vi "Add Channel to Objects.vi"(8 "error in":errorcluster, 9 "Add? (T)":bool=TRUE, 10 "Line Item in":T1, 11 "Objects in":T2) -> (0 "error out":errorcluster, 2 "Line Index":i32)   [LabVIEW 2015, in "TDMS datalogger editor node.lvclass"]
uses:
  TDMS datalogger editor node.lvclass
  <vilib>/NI/DCAF/Tag Editor Core/Table API/Table Manager/object ref.ctl
  <vilib>/NI/DCAF/Tag Editor Core/Configuration Editor/Classes/Engine Parent/Engine Parent Editor Node.lvclass
  <vilib>/NI/DCAF/Tag Editor Core/Configuration Editor/Classes/Module editor node/module editor node.lvclass
  <vilib>/NI/Tag Bus Module Framework/channel/TBM channel.lvclass
  module/configuration/TDMS datalogger configuration.lvclass
  <vilib>/NI/Configuration Framework/serializable configuration/NISE_CEF_serializable configuration.lvclass/NISE_CEF_serializable configuration.ctl
  <vilib>/Utility/LVClass/Get LV Class Name.vi
  <vilib>/NI/Configuration Framework/error generator/NISE_error generator.vi
  <vilib>/NI/Configuration Framework/serializable configuration/NISE_CEF_serializable configuration.lvclass
  <vilib>/NI/DCAF/Tag Editor Core/Table API/Table Manager/Table Manager.lvclass
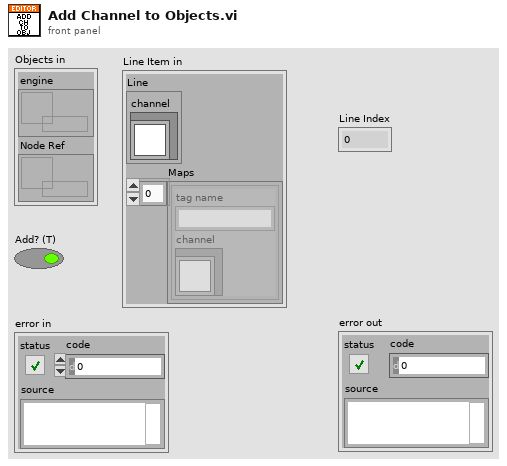
[diagram p1: front panel]
types:
  T1 = cluster{"Line":cluster{"channel":refnum<class "TBM channel.lvclass">}, "Maps":cluster{"tag name":string, "channel":refnum<class "TBM channel.lvclass">}[]}
  T2 = typedef "Table Manager.lvlib/Table Manager.lvclass/object ref.ctl" = cluster{"engine":refnum<data-value>, "Node Ref":refnum<data-value>}
  T3 = cluster{"tag name":string, "channel":refnum<class "TBM channel.lvclass">}[]
  T4 = cluster{"channel":refnum<class "TBM channel.lvclass">}
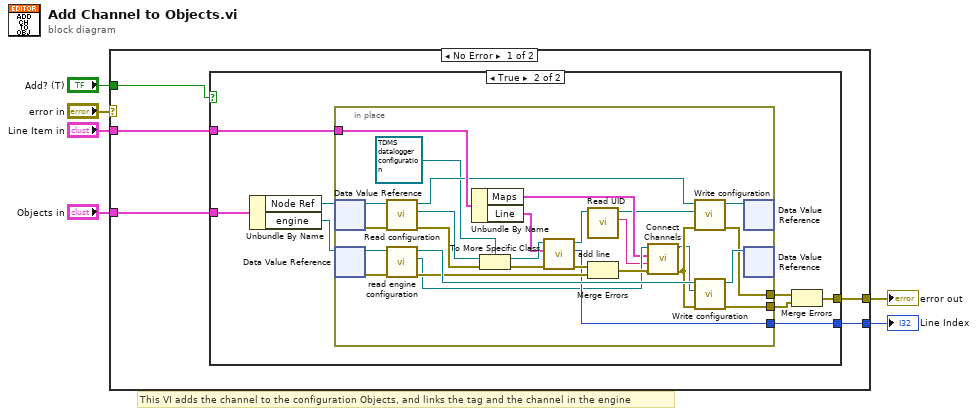
[diagram p0: block diagram]
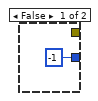
[diagram p2: hidden frame]
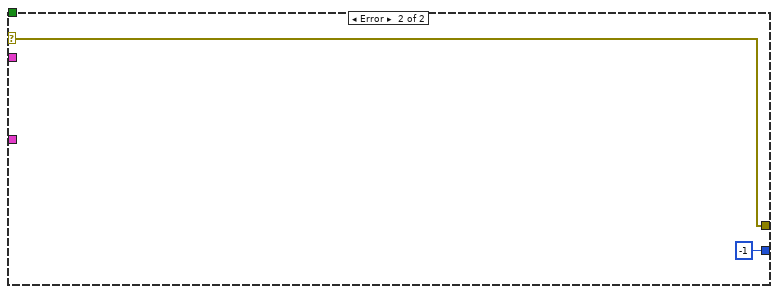
[diagram p3: hidden frame]
diagram:
  # "This VI adds the channel to the configuration Objects, and links the tag and the channel in the engine"
  n1 = case shown="No Error" "error in" {
    selector: "error in" -> [_ w50]
    tunnel: "Objects in" -> [w11 _]
    tunnel: "Line Item in" -> [w10 _]
    tunnel: "Add? (T)" -> [w9 _]
    tunnel: [w8 w50] -> w3
    tunnel: [w7 -1 ("Line Index")] -> w2
    frame No Error {
      n2 = case shown="True" w9 {
        tunnel: [_ w18] -> w8
        tunnel: w10 -> [_ w20]
        tunnel: w11 -> [_ w19]
        tunnel: [-1 ("Line Index") w13] -> w7
        frame False {
        }
        frame True {
          n3 = Unbundle By Name(w19) -> ("Node Ref"=w17:refnum<data-value>, "engine"=w16:refnum<data-value>)
          n4 = in-place {
            in-place-border: w20 -> [w48]
            in-place-border: [w41] -> w15
            in-place-border: [w39] -> w14
            in-place-border: [w29] -> w13
            n5 = in-place-dvr #1(w17) -> (w47:refnum<class "module editor node.lvclass">, w40:errorcluster)
            n6 = in-place-dvr #2(w16) -> (w38:refnum<class "Engine Parent Editor Node.lvclass">, w37:errorcluster)
            n7 = call-dynamic "Read configuration.vi"("error in"=w40, "NISE_CEF_serializable node in"=w47) -> ("error out"=w42:errorcluster, "configuration"=w43:refnum<class "NISE_CEF_serializable configuration.lvclass">, "NISE_CEF_serializable node out"=w46:refnum<class "module editor node.lvclass">)  [unwired: 7 in]
            n8 = call <vilib>:"read engine configuration.vi"("error in"=w37, "Engine Parent Editor Node in"=w38) -> ("error out"=w35:errorcluster, "engine configuration"=w24:refnum<class "engine configuration.lvclass">, "Engine Parent Editor Node out"=w36:refnum<class "Engine Parent Editor Node.lvclass">)  [unwired: 7 in]
            n9 = Unbundle By Name(w48) -> ("Maps"=w23:T3, "Line"=w32:T4)
            n10 = To More Specific Class(target class=refnum<class "TDMS datalogger configuration.lvclass"> refnum ("TDMS datalogger configuration"), reference=w43, error in=w42) -> (specific class reference=w33:refnum<class "TDMS datalogger configuration.lvclass">, error out=w31:errorcluster)
            n11 = call "add line.vi"("error in"=w31, "Line"=w32, "TDMS datalogger configuration in"=w33) -> ("error out"=w30:errorcluster, "Line Index"=w29:i32, "TDMS datalogger configuration out"=w28:refnum<class "TDMS datalogger configuration.lvclass">)  [unwired: 6 in]
            n12 = call <vilib>:"Read UID.vi"("configuration in"=w28) -> ("instance id"=w22:string, "configuration out"=w21:refnum<class "TDMS datalogger configuration.lvclass">)  [unwired: 8 in, 1 out]
            n13 = Merge Errors(w30, w35) -> (w27:errorcluster)
            n14 = call "Connect Channels.vi"("error in (no error)"=w27, "instance id"=w22, "Maps"=w23, "Engine Configuration in"=w24) -> ("error out"=w26:errorcluster, "Engine Configuration out"=w25:refnum<class "engine configuration.lvclass">)  [unwired: 6 in]
            n15 = call-dynamic "Write configuration.vi"("error in"=w26, "configuration"=w21, "NISE_CEF_serializable node in"=w46) -> ("error out"=w39:errorcluster, "NISE_CEF_serializable node out"=w45:refnum<class "module editor node.lvclass">)  [unwired: 7 in]
            n16 = call-dynamic "Write configuration.vi"("error in"=w26, "configuration"=w25, "NISE_CEF_serializable node in"=w36) -> ("error out"=w41:errorcluster, "NISE_CEF_serializable node out"=w44:refnum<class "Engine Parent Editor Node.lvclass">)  [unwired: 7 in]
            n17 = in-place-dvr #1(w45) -> ()  [unwired: 2 out]
            n18 = in-place-dvr #2(w44) -> ()  [unwired: 2 out]
          }
          n19 = Merge Errors(w14, w15) -> (w18:errorcluster)
        }
      }
    }
    frame Error {
    }
  }
  "error out" <- w3
  "Line Index" <- w2
